vi "Stream to AVI Files.vi"() -> ()   [LabVIEW 2023]
doc: "The Stream to AVI Files example shows how to save images to an AVI file when using a grab acquisition. This example uses a grab acquisition which works for all camera formats and image sizes. It is recommended to use the Stream to AVI File (Optimized Performance) example if your camera settings work with a ring acquisition."
uses:
  <vilib>/vision/Avi.llb/IMAQ AVI2 Codec Path.ctl
  SubVIs/Grab Manager Mode.ctl
  <vilib>/vision/Image Controls.llb/IMAQ Image.ctl
  <vilib>/vision/driver/IMAQdx.llb/IMAQdx Buffer Number Mode.ctl
  <vilib>/Utility/High Resolution Relative Seconds.vi
  <vilib>/vision/driver/NI_Vision_Acquisition_Software.lvlib
  <resource>/objmgr/imaqdx.rc
panel:
  in  "Skip Count":u32
  out "Images Saved Per Second":dbl
  out "Images Acquired Per Second":dbl
  in  "Images per AVI":i32=100
  out "Write Speed":dbl(graph) caption="Image File Write Speed"
  in  "Start":bool
  in  "Codec":u16(ring) items=["Microsoft Video 1", "Intel IYUV codec", "Cinepak Codec by Radius", "FF Video Codec 1 (FFV1) (NI Vision)", "Motion JPEG (NI Vision)", "Y800 Uncompressed Grey Scale (NI Vision)", "YUV 4:2:0 Planar (NI Vision)"]
  out "Destination Folder":path
  out "Images Behind":i32
  in  "Number of Images":u32=30
  in  "Camera Name":refnum<k21> caption="IMAQdx Session"
  in  "Stop":bool
  # "Overview: Demonstrates how to stream images to an AVI file when using a grab acquisition.\nRequirements: Vision Acquisition Software\nInstructions:\n1. Select the Camera Name\n2. Run the VI\n3. Select the Codec and click Start.\n4. Increase the Skip Count if Images Behind is greater than 0."
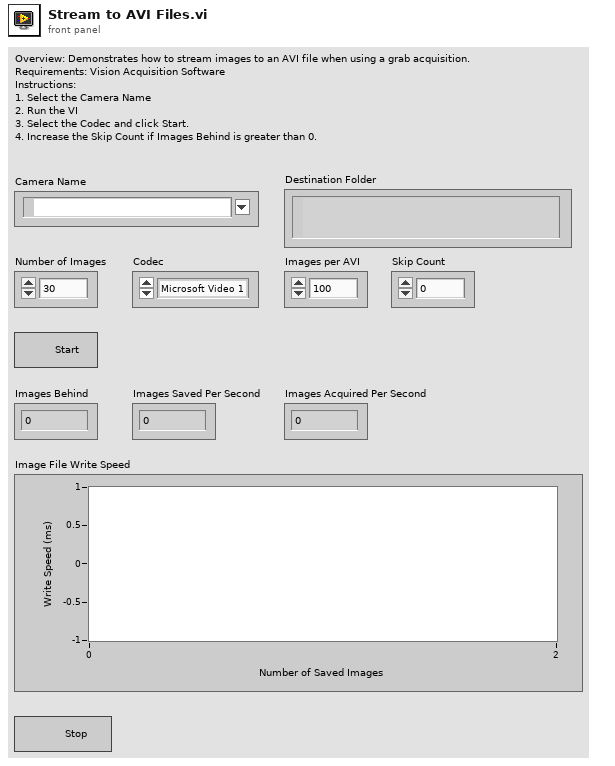
[diagram p1: front panel]
types:
  T1 = typedef "IMAQ AVI2 Codec Path.ctl" = u32
  T2 = typedef "IMAQdx.ctl" = refnum<k21>
  T3 = typedef "IMAQ Image.ctl" = refnum<image>
  T4 = typedef "Grab Manager Mode.ctl" = enum16{"Create Processing Images", "Lock", "Add Acquired Image", "Get Acquired Image", "Unlock", "Dispose Processing Images"}
  T5 = cluster{"Number of Processing Images":u32, "Image Border Size":u32}
  T6 = typedef "NI_Vision_Acquisition_Software.lvlib/IMAQdx Buffer Number Mode.ctl" = enum32{"Next", "Last", "Buffer Number", "Every", "Last New"}
  T7 = typedef "IMAQ AVI2 Refnum.ctl" = refnum<k20>
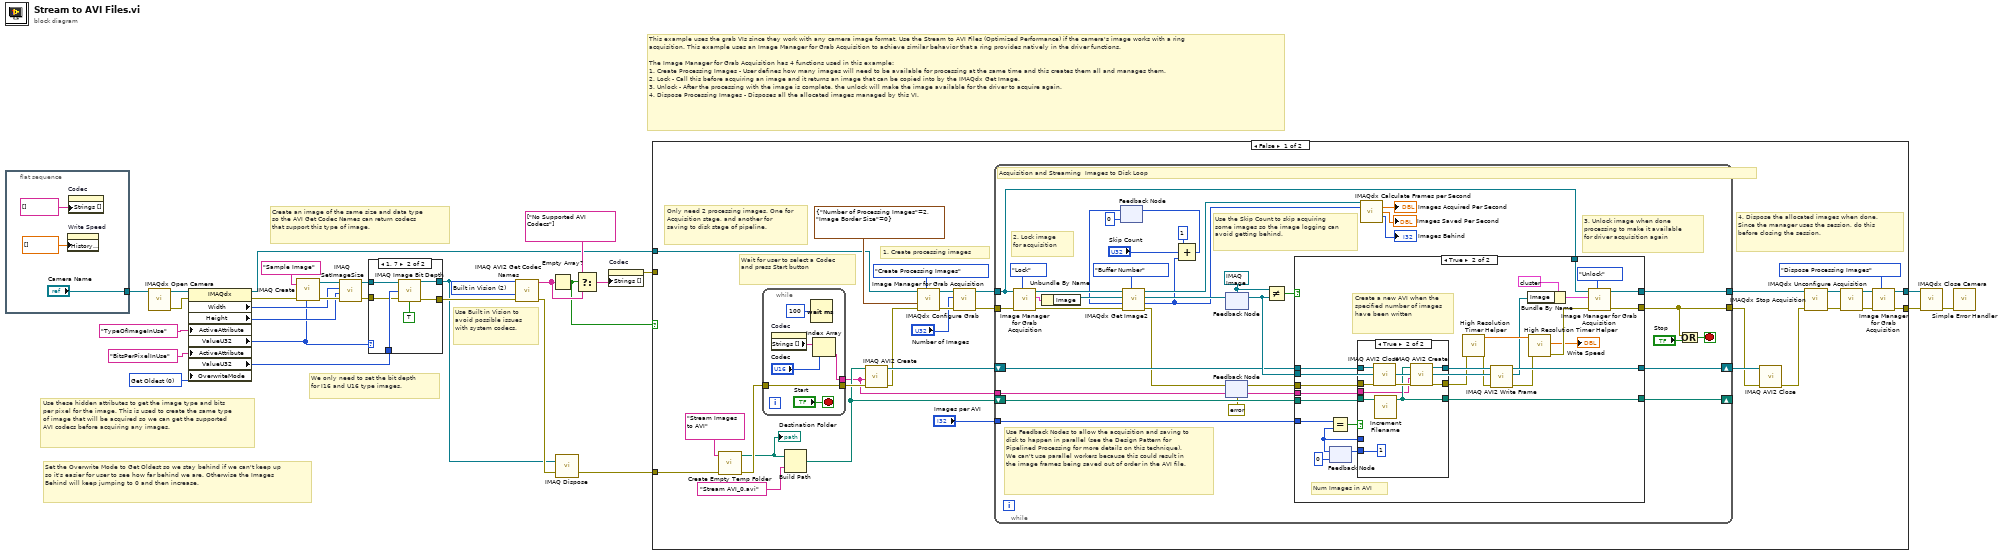
[diagram p0: block diagram]
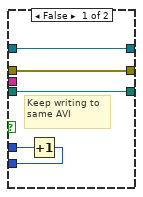
[diagram p3: hidden frame]
diagram:
  w1 = T1 2 items=["Default", "System", "Built in Vision"] ("Codec Source")
  w3 = u32 0 items=["Get Oldest"=0, "Fail"=2, "Get Newest"=3] ("OverwriteMode")
  # "Use Built in Vision to avoid possible issues with system codecs."
  # "This example uses the grab VIs since they work with any camera image format. Use the Stream to AVI Files (Optimized Performance) if the camera's image works with a ring acquisition. This example uses an Image Manager for Grab Acquisition to achieve similar behavior that a ring provides natively in the driver functions.\n\nThe Image Manager for Grab Acquisition has 4 functions used in this example:\n1. Create Processing Images - User defines how many images will need to be available for processing at the same time and this creates them all and manages them.\n2. Lock - Call this before acquiring an image and it returns an image that can be copied into by the IMAQdx Get Image.\n3. Unlock - After the processing with the image is complete, the unlock will make the image available for the driver to acquire again.\n4. Dispose Processing Images - Disposes all the allocated images managed by this VI."
  # "Set the Overwrite Mode to Get Oldest so we stay behind if we can't keep up so it's easier for user to see how far behind we are. Otherwise the Images Behind will keep jumping to 0 and then increase."
  # "Create an image of the same size and data type so the AVI Get Codec Names can return codecs that support this type of image."
  # "Use these hidden attributes to get the image type and bits per pixel for the image. This is used to create the same type of image that will be acquired so we can get the supported AVI codecs before acquiring any images."
  # "We only need to set the bit depth for I16 and U16 type images."
  n1 = flat-sequence {
    tunnel: ["Camera Name"] -> w30
    frame #0 {
      n2 = property on="Write Speed" class="WFChart (strict)"("History Data"=dbl[] []) -> ()  [unwired: 2 in, 2 out]
      n3 = property on="Codec" class="Ring (strict)"("Strings []"=string[] []) -> ()  [unwired: 2 in, 2 out]
    }
  }
  n4 = call <vilib>:"IMAQdx Open Camera.vi"("Session In"=w30) -> ("error out"=w26:errorcluster, "Session Out"=w27:T2)  [unwired: 2 in, 7 out]
  n5 = property class="IMAQdx"(reference=w27, error in=w26, "ActiveAttribute"="TypeOfImageInUse", "ActiveAttribute"="BitsPerPixelInUse", "OverwriteMode"=w3) -> (reference out=w12:T2, error out=w24:errorcluster, "Width"=w20:u32, "Height"=w19:u32, "ValueU32"=w7:u32, "ValueU32"=w10:u32)
  n6 = call "IMAQ Create"("Image Name"="Sample Image", "Image Type"=w7, "error in (no error)"=w24) -> ("New Image"=w21:T3, "error out"=w22:errorcluster)  [unwired: 1 in, 1 out]
  n7 = call "IMAQ SetImageSize"("error in (no error)"=w22, "Y Resolution"=w19, "X Resolution"=w20, "Image"=w21) -> ("error out"=w9:errorcluster, "Image Out"=w8:T3)  [unwired: 1 in]
  n8 = case shown="1, 7" w7 {
    tunnel: [w34 w41] -> w13
    tunnel: w10 -> [_ w40]
    tunnel: w9 -> [w34 w39]
    tunnel: w8 -> [w35 w37]
    tunnel: [w35 w36] -> w4
    frame 0, Default {
    }
    frame 1, 7 {
      n9 = call "IMAQ Image Bit Depth"("Image"=w37, "Bit Depth (0)"=w40, "error in (no error)"=w39, "Get/Set Bit Depth? (Set)"=TRUE) -> ("Image Out"=w36:T3, "error out"=w41:errorcluster)  [unwired: 9 in, 1 out]
    }
  }
  n10 = call "IMAQ AVI2 Get Codec Names"("error in (no error)"=w13, "Codec Source"=w1, "Image"=w4) -> ("error out"=w6:errorcluster, "Codec Names"=w18:string[])  [unwired: 7 in]
  n11 = Empty Array?(array=w18) -> (empty?=w14:bool)
  n12 = call "IMAQ Dispose"("Image"=w4, "error in (no error)"=w6) -> ("error out"=w5:errorcluster)  [unwired: 4 in]
  n13 = Select(t=string[] ["No Supported AVI Codecs"], s=w14, f=w18) -> (s? t:f=w16:string[])
  n14 = property on="Codec" class="Ring (strict)"("Strings []"=w16) -> (error out=w15:errorcluster)  [unwired: 2 in, 1 out]
  n15 = case shown="False" w14 {
    tunnel: [w43 w157] -> w29
    tunnel: [w44 w158] -> w28
    tunnel: w12 -> [w49 w158]
    tunnel: w5 -> [w52 w157]
    tunnel: w15 -> [_ _]
    frame False {
      # "4. Dispose the allocated images when done. Since the manager uses the session, do this before closing the session."
      # "1. Create processing images"
      # "Only need 2 processing images. One for Acquisition stage, and another for saving to disk stage of pipeline."
      # "Wait for user to select a Codec and press Start button"
      n16 = call "Create Empty Temp Folder.vi"("error in (no error)"=w52, "Folder Name"="Stream Images to AVI") -> ("error out"=w67:errorcluster, "Empty Temp Folder"=w60:path)  [unwired: 8 in]
      "Destination Folder" <- w60
      n17 = while {
        tunnel: w67 -> [w155]
        tunnel: [w155] -> w66
        tunnel: [w152] -> w57
        stop <- "Start" stop-if-true
        n18 = property on="Codec" class="Ring (strict)"() -> ("Strings []"=w153:string[])  [unwired: 2 in, 2 out]
        n19 = Wait (ms)(milliseconds to wait=u32 100) -> ()  [unwired: 1 out]
        n20 = Index Array(array=w153, index="Codec") -> (element=w152:string)
      }
      n21 = Build Path(base path=w60, name or relative path="Stream AVI_0.avi") -> (appended path=w58:path)
      n22 = call "IMAQ AVI2 Create"("error in (no error)"=w66, "Codec"=w57, "AVI Path"=w58) -> ("error out"=w48:errorcluster, "AVI Refnum"=w61:T7)  [unwired: 7 in]
      n23 = call "Image Manager for Grab Acquisition.vi"("Mode"=Grab_Manager_Mode."Create Processing Images", "error in (no error)"=w48, "Init Settings"=T5 {"Number of Processing Images"=2, "Image Border Size"=0}, "Session In"=w49) -> ("error out"=w51:errorcluster, "Session Out"=w50:T2)  [unwired: 4 in, 2 out]
      n24 = call <vilib>:"IMAQdx Configure Grab.vi"("error in"=w51, "Number of Buffers"="Number of Images", "Session In"=w50) -> ("error out"=w55:errorcluster, "Session Out"=w56:T2)  [unwired: 7 in]
      n25 = while {
        tunnel: w55 -> [w89]
        tunnel: w56 -> [w90]
        tunnel: [w104] -> w69
        tunnel: [w97] -> w64
        shift-right: [w105] -> w65
        shift-left: w61 -> [w96]
        tunnel: "Images per AVI" -> [w92]
        shift-right: [w93] -> _
        shift-left: w58 -> [w94]
        tunnel: w57 -> [w95]
        stop <- w99 stop-if-true
        w102 = T3 refnum ("Image Out")
        # "3. Unlock image when done processing to make it available for driver acquisition again"
        # "2. Lock image for acquisition"
        # "Use the Skip Count to skip acquiring some images so the image logging can avoid getting behind."
        # "Use Feedback Nodes to allow the acquisition and saving to disk to happen in parallel (see the Design Pattern for Pipelined Processing for more details on this technique). We can't use parallel workers because this could result in the image frames being saved out of order in the AVI file."
        # "Acquisition and Streaming  Images to Disk Loop"
        n26 = call "Image Manager for Grab Acquisition.vi"("Mode"=Grab_Manager_Mode."Lock", "error in (no error)"=w89, "Session In"=w90) -> ("error out"=w86:errorcluster, "Image Settings Out"=w84:cluster{"Image":T3, "Buffer Number":u32}, "Session Out"=w87:T2)  [unwired: 5 in, 1 out]
        n27 = Unbundle By Name(w84) -> ("Image"=w83:T3)
        n28 = feedback #1(u32 0) -> (w79:u32)
        n29 = call <vilib>:"IMAQdx Get Image2.vi"("Buffer Number Mode (Next)"=IMAQdx_Buffer_Number_Mode."Buffer Number", "error in"=w86, "Buffer Number In"=w79, "Image In"=w83, "Session In"=w87) -> ("error out"=w82:errorcluster, "Buffer Number Out"=w75:u32, "Image Out"=w80:T3, "Session Out"=w81:T2)  [unwired: 3 in]
        n30 = Compound Arithmetic op=ADD(u32 1, "Skip Count", w75) -> (w74:u32)
        n31 = feedback-in #1(w74) -> ()
        n32 = feedback-in #2(w82) -> ()
        n33 = feedback #2(errorcluster {"status"=FALSE, "code"=0, "source"=""} ("error out")) -> (w103:errorcluster)
        n34 = feedback-in #3(w80) -> ()
        n35 = feedback #3(w102) -> (w100:T3)
        n36 = Not Equal?(x=w102, y=w100) -> (x != y?=w101:bool)
        n37 = case shown="True" w101 {
          tunnel: w96 -> [w108 w131]
          tunnel: w100 -> [_ w125]
          tunnel: w103 -> [w109 w130]
          tunnel: [w108 w136] -> w105
          tunnel: [w110 w119] -> w104
          tunnel: w90 -> [w110 w116]
          tunnel: [w109 w118] -> w97
          tunnel: w95 -> [_ w129]
          tunnel: w94 -> [w107 w128]
          tunnel: [w107 w126] -> w93
          tunnel: w92 -> [_ w124]
          frame False {
            # "First iteration doesn't have valid image for this pipelined stage."
          }
          frame True {
            # "Create a new AVI when the specified number of images have been written"
            # "Num Images in AVI"
            n38 = feedback #4(0) -> (w135:i32)
            n39 = Equal?(x=w124, y=w135) -> (x = y?=w132:bool)
            n40 = case shown="True" w132 {
              tunnel: [w140 1] -> w134
              tunnel: w135 -> [w141 _]
              tunnel: w131 -> [w139 w148]
              tunnel: [w139 w145] -> w127
              tunnel: w128 -> [w137 w149]
              tunnel: w130 -> [w138 w147]
              tunnel: [w138 w144] -> w123
              tunnel: [w137 w143] -> w126
              tunnel: w129 -> [_ w142]
              frame False {
                # "Keep writing to same AVI"
                n41 = Increment(x=w141) -> (x+1=w140:i32)
              }
              frame True {
                n42 = call "IMAQ AVI2 Close"("error in (no error)"=w147, "AVI Refnum"=w148) -> ("error out"=w146:errorcluster)  [unwired: 9 in]
                n43 = call "Increment Filename.vi"("Path In"=w149) -> ("Incremented Path Out"=w143:path)  [unwired: 10 in]
                n44 = call "IMAQ AVI2 Create"("error in (no error)"=w146, "Codec"=w142, "AVI Path"=w143) -> ("error out"=w144:errorcluster, "AVI Refnum"=w145:T7)  [unwired: 7 in]
              }
            }
            n45 = feedback-in #4(w134) -> ()
            n46 = call "High Resolution Timer Helper.vi"("error in (no error)"=w123) -> ("error out"=w122:errorcluster, "Current Time"=w120:dbl)  [unwired: 8 in, 1 out]
            n47 = call "IMAQ AVI2 Write Frame"("error in (no error)"=w122, "Image"=w125, "AVI Refnum"=w127) -> ("error out"=w121:errorcluster, "Image Out (duplicate)"=w113:T3, "AVI Refnum (duplicate)"=w136:T7)  [unwired: 6 in]
            n48 = Bundle By Name(cluster=cluster{"Image":T3, "Buffer Number":u32} {"Image"=refnum, "Buffer Number"=0} ("Image Settings In"), "Image"=w113) -> (w112:cluster{"Image":T3, "Buffer Number":u32})
            n49 = call "High Resolution Timer Helper.vi"("error in (no error)"=w121, "Previous Time"=w120) -> ("error out"=w117:errorcluster, "Time Difference (ms)"=→"Write Speed":dbl)  [unwired: 7 in, 1 out]
            n50 = call "Image Manager for Grab Acquisition.vi"("Mode"=Grab_Manager_Mode."Unlock", "error in (no error)"=w117, "Image Settings In"=w112, "Session In"=w116) -> ("error out"=w118:errorcluster, "Session Out"=w119:T2)  [unwired: 4 in, 2 out]
          }
        }
        n51 = call <vilib>:"IMAQdx Calculate Frames per Second.vi"("Session In"=w81, "Buffer Number"=w75) -> ("Acquired Frames per Second"=→"Images Acquired Per Second":dbl, "Processed Frames per Second"=→"Images Saved Per Second":dbl, "Images Behind"=→"Images Behind":i32)  [unwired: 7 in, 4 out]
        n52 = Or(x=w97, y="Stop") -> (x .or. y?=w99:bool)
      }
      n53 = call "IMAQ AVI2 Close"("error in (no error)"=w64, "AVI Refnum"=w65) -> ("error out"=w63:errorcluster)  [unwired: 9 in]
      n54 = call <vilib>:"IMAQdx Stop Acquisition.vi"("error in"=w63, "Session In"=w69) -> ("error out"=w70:errorcluster, "Session Out"=w71:T2)  [unwired: 8 out]
      n55 = call <vilib>:"IMAQdx Unconfigure Acquisition.vi"("error in"=w70, "Session In"=w71) -> ("error out"=w47:errorcluster, "Session Out"=w46:T2)  [unwired: 8 out]
      n56 = call "Image Manager for Grab Acquisition.vi"("Mode"=Grab_Manager_Mode."Dispose Processing Images", "error in (no error)"=w47, "Session In"=w46) -> ("error out"=w43:errorcluster, "Session Out"=w44:T2)  [unwired: 5 in, 2 out]
    }
    frame True {
      # "No valid AVI Codecs for the image size and image type."
    }
  }
  n57 = call <vilib>:"IMAQdx Close Camera.vi"("error in"=w29, "Session In"=w28) -> ("error out"=w2:errorcluster)  [unwired: 9 out]
  n58 = call <vilib>:"Simple Error Handler.vi"("error in (no error)"=w2) -> ()  [unwired: 4 in, 5 out]
